vi "TEST_RealMeasure.vi"() -> ()   [LabVIEW 2020]
uses:
  ProligentResultProcessor/Measure/RangeMeasureLimit/ComparisonType.ctl
  ProligentResultProcessor/Datawarehouse/Datawarehouse.lvclass
  ProligentResultProcessor/ProcessRun/ProcessRun.lvclass
  ProligentResultProcessor/OperationRun/OperationRun.lvclass
  ProligentResultProcessor/SequenceRun/SequenceRun/SequenceRun.lvclass
  ProligentResultProcessor/StepRun/StepRun/StepRun.lvclass
  ProligentResultProcessor/Measure/RealMeasure/RealMeasure.lvclass
  ProligentResultProcessor/Measure/RangeMeasureLimit/RangeMeasureLimit.lvclass
panel:
  out "error out":errorcluster
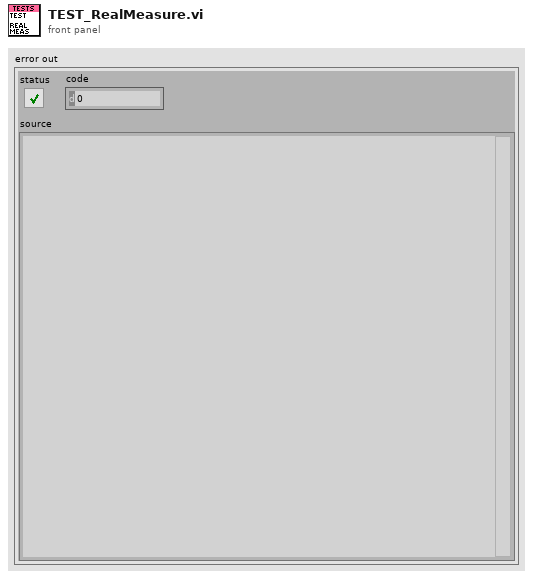
[diagram p1: front panel]
types:
  T1 = typedef "ProligentResultProcessor.lvlib/RangeMeasureLimit.lvclass/ComparisonType.ctl" = enum16{"LowerBound <= X <= HigherBound", "LowerBound < X <= HigherBound", "LowerBound <= X < HigherBound", "LowerBound < X < HigherBound", "LowerBound <= X", "LowerBound < X", "X <= HigherBound", "X < HigherBound", "X == HigherBound", "X != HigherBound", "X <= LowerBound OR HigherBound <= X", "X < LowerBound OR HigherBound <= X", "X <= LowerBound OR HigherBound < X", "X < LowerBound OR HigherBound < X"}
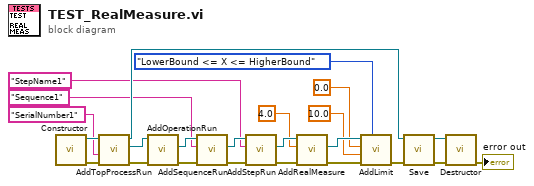
[diagram p0: block diagram]
diagram:
  n1 = call "Constructor.vi"() -> ("error out"=w23:errorcluster, "Datawarehouse"=w24:refnum<class "Datawarehouse.lvclass">)  [unwired: 10 in]
  n2 = call "AddTopProcessRun.vi"("error in"=w23, "ProductUnitIdentifier"="SerialNumber1" ("OperationName (Generic_Operation)"), "Datawarehouse in"=w24) -> ("error out"=w17:errorcluster, "TopProcessRun"=w20:refnum<class "ProcessRun.lvclass">, "Datawarehouse out"=w22:refnum<class "Datawarehouse.lvclass">)  [unwired: 6 in]
  n3 = call "AddOperationRun.vi"("error in"=w17, "ProcessRun in"=w20) -> ("error out"=w19:errorcluster, "OperationRun"=w18:refnum<class "OperationRun.lvclass">)  [unwired: 7 in, 1 out]
  n4 = call "AddSequenceRun.vi"("error in"=w19, "SequenceFullName"="Sequence1", "OperationRun in"=w18) -> ("error out"=w16:errorcluster, "SequenceRun"=w15:refnum<class "SequenceRun.lvclass">)  [unwired: 6 in, 1 out]
  n5 = call "AddStepRun.vi"("error in"=w16, "StepName"="StepName1", "SequenceRun in"=w15) -> ("error out"=w13:errorcluster, "StepRun"=w14:refnum<class "StepRun.lvclass">)  [unwired: 6 in, 1 out]
  n6 = call "AddRealMeasure.vi"("error in"=w13, "Value"=4.0, "StepRun in"=w14) -> ("error out"=w9:errorcluster, "RealMeasure"=w10:refnum<class "RealMeasure.lvclass">)  [unwired: 6 in, 1 out]
  n7 = call "AddLimit.vi"("ComparisonType"=ComparisonType."LowerBound <= X <= HigherBound", "error in"=w9, "HigherBond"=10.0, "LowerBound"=0.0, "RealMeasure in"=w10) -> ("error out"=w8:errorcluster)  [unwired: 4 in, 2 out]
  n8 = call "Save.vi"("error in"=w8, "Datawarehouse in"=w22) -> ("error out"=w12:errorcluster, "Datawarehouse out"=w21:refnum<class "Datawarehouse.lvclass">)  [unwired: 8 in]
  n9 = call "Destructor.vi"("error in"=w12, "Datawarehouse"=w21) -> ("error out"=→"error out":errorcluster)  [unwired: 9 in]
